vi "DAC_Init.vi"(8 "error in (no error)":errorcluster) -> (0 "error out":errorcluster)   [LabVIEW 2012]
panel:
  out "Device Mask":u32 format="%032b"
  out "Counters":u32 format="%.0g"
  out "DIO Bytes":u32 format="%.0g"
  out "Board Name":string
  out "Product ID":u32 format="%.0x"
  in  "DeviceIndex":i32
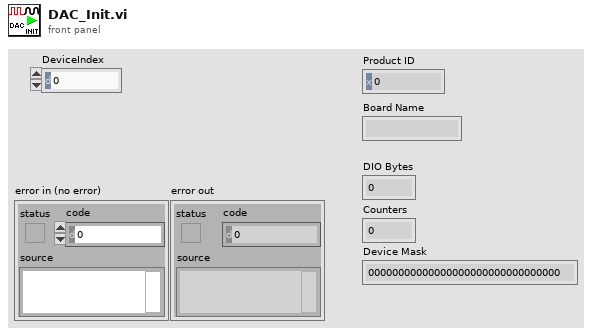
[diagram p1: front panel]
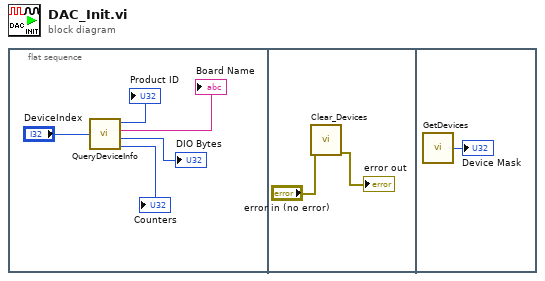
[diagram p0: block diagram]
diagram:
  n1 = flat-sequence {
    frame #0 {
      n2 = call "QueryDeviceInfo.vi"("DeviceIndex"="DeviceIndex") -> ("Product ID"=→"Product ID":u32, "Board Name"=→"Board Name":string, "DIO Bytes"=→"DIO Bytes":u32, "Counters"=→"Counters":u32)
    }
    frame #1 {
      n3 = call "Clear_Devices.vi"("error in (no error)"="error in (no error)") -> ("error out"=→"error out":errorcluster)  [unwired: 10 in]
    }
    frame #2 {
      n4 = call "GetDevices.vi"() -> ("Device Mask"=→"Device Mask":u32)
    }
  }
